vi "VIScriptingTest.vi"(10 "Mouse Coords":T1, 11 "New Node Name":string) -> (2 "Canceled":bool, 3 "Attributes":string[][](array[string]))   [LabVIEW 2017]
uses:
  <vilib>/Utility/miscctls.llb/LVPoint32TypeDef.ctl
  <vilib>/Utility/Data Type/NI_Data Type.lvlib
panel:
  out "Array":variant[](array[variant])
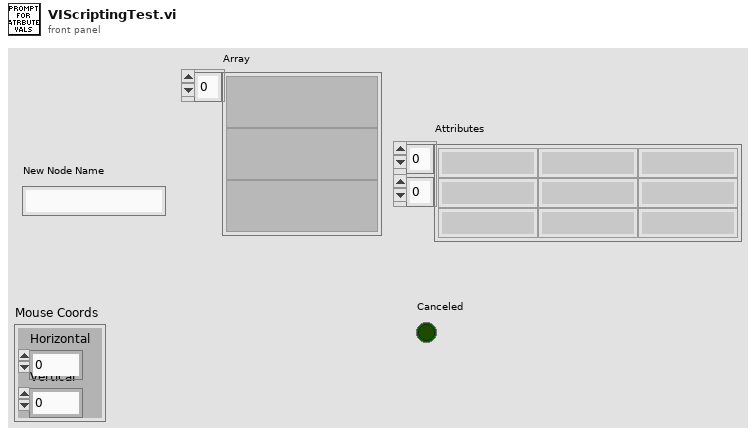
[diagram p1: front panel]
types:
  T1 = typedef "LVPoint32TypeDef.ctl" = cluster{"Horizontal":i32, "Vertical":i32}
  T2 = cluster{"Horizontal":i32, "Vertical":i32, "Horizontal":i32, "Vertical":i32}
  T3 = typedef "NI_Data Type.lvlib/Data Type.ctl" = enum8{"Invalid Type", "Void", "I8", "I16", "I32", "I64", "U8", "U16", "U32", "U64", "Single Float", "Double Float", "Extended Float", "Single Complex", "Double Complex", "Extended Complex", "Enum U8", "Enum U16", "Enum U32", "Enum U64", "Single Float With Unit", "Double Float With Unit", "Extended Float With Unit", "Single Complex with Unit", "Double Complex with Unit", "Extended Complex with Unit", "Boolean", "String", "Path", "Picture", "Tag", "Array", "Cluster", "Variant", "LV Variant", "Waveform", "Timestamp", "Digital Waveform", "Digital Data", "ExpressData", "Refnum", "External Data", "VI", "Poly VI", "LabVIEW Class Instance", "Fixed Point"}
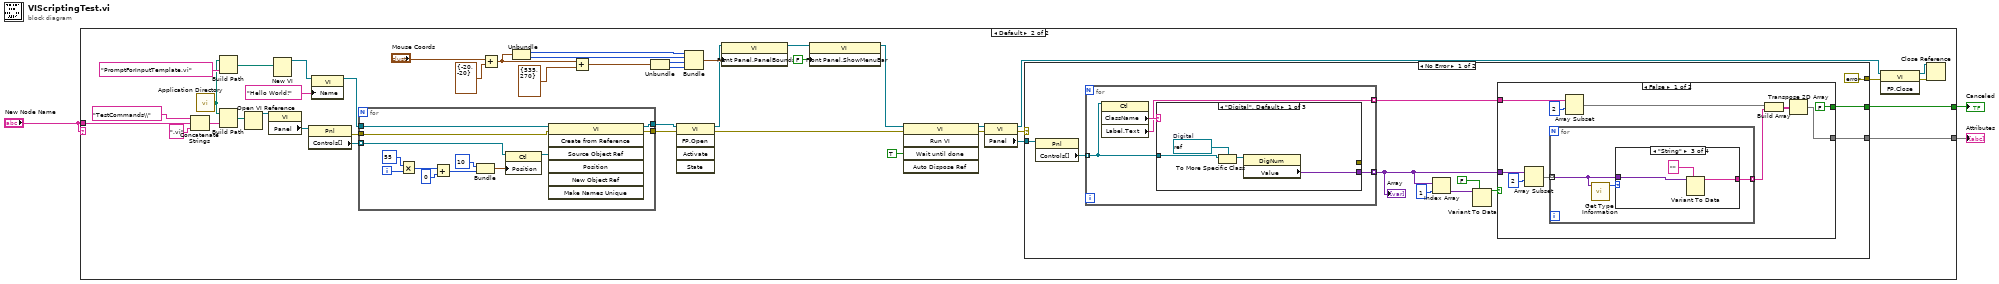
[diagram p0: block diagram]
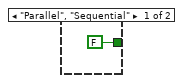
[diagram p2: hidden frame]
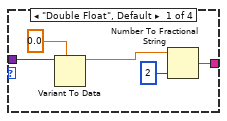
[diagram p3: hidden frame]
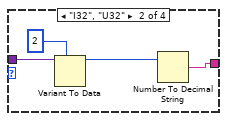
[diagram p4: hidden frame]
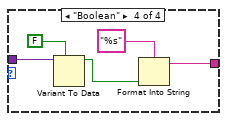
[diagram p5: hidden frame]
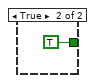
[diagram p6: hidden frame]
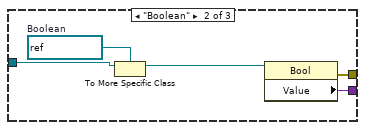
[diagram p7: hidden frame]
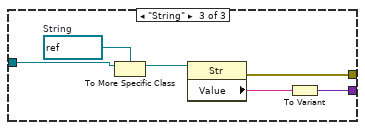
[diagram p8: hidden frame]
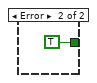
[diagram p9: hidden frame]
diagram:
  n1 = case shown="Default" "New Node Name" {
    tunnel: "New Node Name" -> [_ w31]
    tunnel: [FALSE ("Canceled") w24] -> w2
    tunnel: [_ w23] -> w1
    frame "Parallel", "Sequential" {
    }
    frame Default {
      n2 = Concatenate Strings("TestCommands\\" ("string"), w31, ".vi" ("string")) -> (w28:string)
      n3 = call <vilib>:"Application Directory.vi"() -> ("Application Directory"=w27:path)
      n4 = Build Path(base path=w27, name or relative path="PromptForInputTemplate.vi") -> (appended path=w32:path)
      n5 = Build Path(base path=w27, name or relative path=w28) -> (appended path=w26:path)
      n6 = Open VI Reference(vi path=w26) -> (vi reference=w8:refnum<vi>)  [unwired: 5 in, 1 out]
      n7 = property class="VI"(reference=w8) -> ("Panel"=w42:refnum<vi>)  [unwired: 1 in, 2 out]
      n8 = New VI(10:w32) -> (3:w37:refnum<vi>)  [unwired: 6 in, 1 out]
      n9 = property class="Pnl"(reference=w42) -> (error out=w44:errorcluster, "Controls[]"=w45:refnum<vi>[])  [unwired: 1 in, 1 out]
      n10 = property class="VI"(reference=w37, "Name"="Hello World!" ("VI Name")) -> (reference out=w43:refnum<vi>)  [unwired: 1 in, 1 out]
      n11 = for {
        tunnel: w43 -> [w122]
        tunnel: w44 -> [w121]
        tunnel: w45 -> [w110] mode=indexing
        tunnel: [w120] -> w46
        tunnel: [w119] -> w47
        i -> [w118]
        n12 = Multiply(x=55, y=w118) -> (x*y=w116:i32)
        n13 = Add(x=w116, y=0) -> (x+y=w113:i32)
        n14 = Bundle("y"=10, w113) -> (w111:cluster{"y":i32, i32})  [unwired: 1 in]
        n15 = property class="Ctl"(reference=w110, "Position"=w111) -> (reference out=w114:refnum<vi>)  [unwired: 1 in, 1 out]
        n16 = invoke class="VI" method="Create from Reference"(reference=w122, error in=w121, "Source Object Ref"=w114) -> (reference out=w120:refnum<vi>, error out=w119:errorcluster)  [unwired: 4 in, 5 out]
      }
      n17 = Add(x="Mouse Coords", y=T1 {"Horizontal"=-20, "Vertical"=-20}) -> (x+y=w10:T1)
      n18 = Unbundle(w10) -> ("Horizontal"=w17:i32, "Vertical"=w16:i32)
      n19 = Add(x=w10, y=cluster{"Left":i16, "Top":i16} {"Left"=535, "Top"=270} ("Front Panel Window:Panel Bounds")) -> (x+y=w19:T1)
      n20 = Unbundle(w19) -> ("Horizontal"=w15:i32, "Vertical"=w14:i32)
      n21 = invoke class="VI" method="FP.Open"(reference=w46, error in=w47) -> (reference out=w7:refnum<vi>, error out=w36:errorcluster)  [unwired: 3 in, 3 out]
      n22 = Bundle("Horizontal"=w17, "Vertical"=w16, "Horizontal"=w15, "Vertical"=w14) -> (w13:T2)  [unwired: 1 in]
      n23 = property class="VI"(reference=w7, "Front Panel.PanelBounds"=w13) -> (reference out=w6:refnum<vi>)  [unwired: 1 in, 1 out]
      n24 = property class="VI"(reference=w6, "Front Panel.ShowMenuBar"=FALSE ("Front Panel Window:Show Menu Bar")) -> (reference out=w5:refnum<vi>)  [unwired: 1 in, 1 out]
      n25 = invoke class="VI" method="Run VI"(reference=w5, error in=w36, "Wait until done"=TRUE ("Wait Until Done")) -> (reference out=w38:refnum<vi>, error out=w39:errorcluster)  [unwired: 2 in, 3 out]
      n26 = property class="VI"(reference=w38, error in=w39) -> (reference out=w41:refnum<vi>, error out=w25:errorcluster, "Panel"=w40:refnum<vi>)
      n27 = case shown="No Error" w25 {
        tunnel: w40 -> [w57 _]
        tunnel: [w53 TRUE ("Canceled")] -> w24
        tunnel: [w50 _] -> w23
        tunnel: [errorcluster {"status"=FALSE, "code"=0, "source"=""} ("error constant") _] -> w20
        frame No Error {
          n28 = property class="Pnl"(reference=w57) -> ("Controls[]"=w58:refnum<vi>[])  [unwired: 1 in, 2 out]
          n29 = for {
            tunnel: w58 -> [w93] mode=indexing
            tunnel: [w91] -> w52 mode=indexing
            tunnel: [w90] -> w49 mode=indexing
            n30 = property class="Ctl"(reference=w93) -> ("ClassName"=w92:string, "Label.Text"=w90:string)  [unwired: 1 in, 2 out]
            n31 = case shown="\"Digital\", Default" w92 {
              tunnel: [_ w100 w106] -> _
              tunnel: w93 -> [w95 w99 w105]
              tunnel: [w94 w98 w103] -> w91
              frame "Digital", Default {
                w97 = refnum<vi> refnum  # Digital
                n32 = To More Specific Class(target class=w97, reference=w95) -> (specific class reference=w96:refnum<vi>)  [unwired: 1 in, 1 out]
                n33 = property class="DigNum"(reference=w96) -> ("Value"=w94:variant)  [unwired: 1 in, 2 out]
              }
              frame "Boolean" {
                w102 = refnum<vi> refnum  # Boolean
                n34 = To More Specific Class(target class=w102, reference=w99) -> (specific class reference=w101:refnum<vi>)  [unwired: 1 in, 1 out]
                n35 = property class="Bool"(reference=w101) -> (error out=w100:errorcluster, "Value"=w98:variant)  [unwired: 1 in, 1 out]
              }
              frame "String" {
                w108 = refnum<vi> refnum  # String
                n36 = To More Specific Class(target class=w108, reference=w105) -> (specific class reference=w107:refnum<vi>)  [unwired: 1 in, 1 out]
                n37 = property class="Str"(reference=w107) -> (error out=w106:errorcluster, "Value"=w104:string)  [unwired: 1 in, 1 out]
                n38 = To Variant(anything=w104) -> (Variant=w103:variant)
              }
            }
          }
          "Array" <- w52
          n39 = Index Array(array=w52, index=1) -> (element=w56:variant)
          n40 = Variant To Data(type=FALSE, Variant=w56) -> (data=w54:bool)  [unwired: 1 in, 1 out]
          n41 = case shown="False" w54 {
            tunnel: [FALSE ("Wait Until Done") TRUE ("Wait Until Done")] -> w53
            tunnel: w52 -> [w67 _]
            tunnel: [w59 _] -> w50
            tunnel: w49 -> [w62 _]
            frame False {
              n42 = Array Subset(array=w67, index=2) -> (w65:variant[])  [unwired: 1 in]
              n43 = for {
                tunnel: w65 -> [w70] mode=indexing
                tunnel: [w69] -> w64 mode=indexing
                n44 = call <vilib>:"Get Type Information.vi"("Variant"=w70) -> ("Type"=w71:T3)  [unwired: 6 in, 4 out]
                n45 = case shown="\"String\"" w71 {
                  tunnel: w70 -> [w74 w79 w83 w88]
                  tunnel: [w72 w78 w81 w86] -> w69
                  frame "Double Float", Default {
                    n46 = Variant To Data(type=0.0, Variant=w74) -> (data=w76:dbl)  [unwired: 1 in, 1 out]
                    n47 = Number To Fractional String(number=w76, precision (6)=i16 2) -> (F-format string=w72:string)  [unwired: 2 in]
                  }
                  frame "I32", "U32" {
                    n48 = Variant To Data(type=i16 2 ("precision (6)"), Variant=w79) -> (data=w80:i16)  [unwired: 1 in, 1 out]
                    n49 = Number To Decimal String(number=w80) -> (decimal integer string=w78:string)  [unwired: 1 in]
                  }
                  frame "String" {
                    n50 = Variant To Data(type="", Variant=w83) -> (data=w81:string)  [unwired: 1 in, 1 out]
                  }
                  frame "Boolean" {
                    n51 = Variant To Data(type=FALSE ("Wait Until Done"), Variant=w88) -> (data=w84:bool)  [unwired: 1 in, 1 out]
                    n52 = Format Into String(format string="%s", w84) -> (resulting string=w86:string)  [unwired: 2 in, 1 out]
                  }
                }
              }
              n53 = Array Subset(array=w62, index=2) -> (w61:string[])  [unwired: 1 in]
              n54 = Build Array(w61, w64) -> (w60:string[][])
              n55 = Transpose 2D Array(2D array=w60) -> (transposed array=w59:string[][])
            }
            frame True {
            }
          }
        }
        frame Error {
        }
      }
      n56 = invoke class="VI" method="FP.Close"(reference=w41, error in=w20) -> (reference out=w22:refnum<vi>, error out=w21:errorcluster)  [unwired: 1 in, 1 out]
      n57 = Close Reference(reference=w22, error in (no error)=w21) -> ()  [unwired: 1 out]
    }
  }
  "Attributes" <- w1
  "Canceled" <- w2
